vi "Unlock_project_folder.vi"() -> ()   [LabVIEW 2023]
uses:
  <vilib>/Utility/error.llb/Trim Whitespace One-Sided.vi
panel:
  out "status":string
  in  "stop":bool
  in  "File types":string="*.vi,*.vit,*.vim,*.ctl,*.ctt,*.lvlib,*.lvclass,*.xctl,*.xnode" caption="File types (comma separated)"
  out "File":path
  out "Slide":dbl(slide) scale=0.0..1.0
  out "Icon":picture
  in  "Output folder":path
  in  "Locked project folder":path
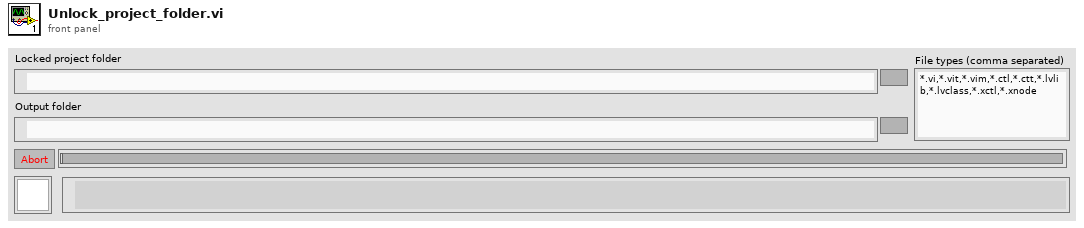
[diagram p1: front panel]
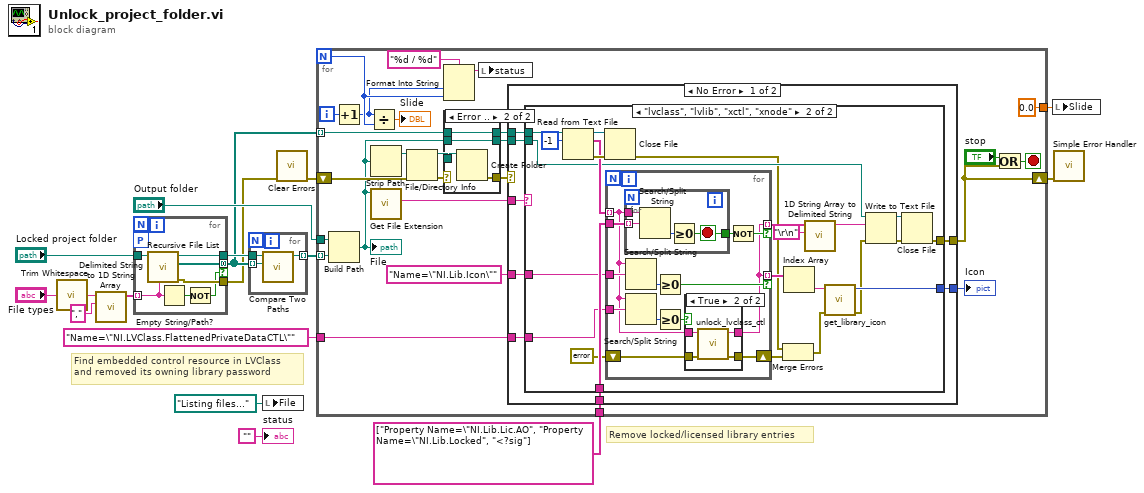
[diagram p0: block diagram]
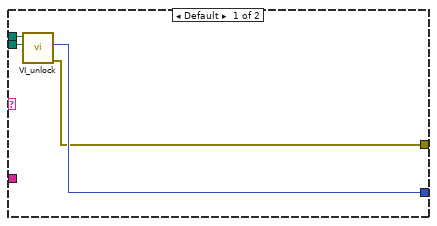
[diagram p3: hidden frame]
diagram:
  # "Remove locked/licensed library entries"
  # "Find embedded control resource in LVClass\nand removed its owning library password"
  n1 = call <vilib>:"Trim Whitespace.vi"("string"="File types") -> ("trimmed string"=w4:string)  [unwired: 1 in]
  n2 = call <vilib>:"Delimited String to 1D String Array.vi"("delimiter"="," ("delimiter (Tab)"), "delimited string"=w4) -> ("string array"=w3:string[])  [unwired: 9 in]
  n3 = for {
    tunnel: w3 -> [w20] mode=indexing
    workers-P: _ -> [_]
    tunnel: "Locked project folder" -> [w24]
    tunnel: [w23] -> w8 mode=concatenating if=w18
    tunnel: [w22] -> w7
    tunnel: [w21] -> w9
    n4 = call <vilib>:"Recursive File List.vi"("pattern"=w20, "Folder Path"=w24) -> ("error out"=w22:errorcluster, "All Files in Dir"=w23:path[], "dup Folder Path"=w21:path)  [unwired: 5 in, 2 out]
    n5 = Empty String/Path?(string/path=w20) -> (empty?=w19:bool)
    n6 = Not(x=w19) -> (.not. x?=w18:bool)
  }
  n7 = for {
    tunnel: w8 -> [w26] mode=indexing
    tunnel: w9 -> [w25]
    tunnel: [w27] -> w15 mode=indexing
    n8 = call <vilib>:"Compare Two Paths.vi"("Path 2"=w26, "Path 1"=w25) -> ("Relative Path from 1 to 2"=w27:path)  [unwired: 6 in, 3 out]
  }
  n9 = local write "File"(path "Listing files..." ("File")) -> ()
  n10 = call <vilib>:"Clear Errors.vi"("error in (no error)"=w7) -> ("error out"=w6:errorcluster)  [unwired: 5 in, 1 out]
  n11 = for {
    N -> [w31]
    tunnel: w8 -> [w39] mode=indexing
    tunnel: "Output folder" -> [w53]
    shift-right: [w34] -> w17
    shift-left: w6 -> [w48]
    tunnel: string[] ["Property Name=\"NI.Lib.Lic.AO", "Property Name=\"NI.Lib.Locked", "<?sig"] -> [w45]
    tunnel: w15 -> [w44] mode=indexing
    tunnel: "Name=\"NI.LVClass.FlattenedPrivateDataCTL\"" ("search string/char (-)") -> [w42]
    tunnel: [0.0] -> w12
    i -> [w50]
    stop <- w33 stop-if-true
    n12 = Build Path(base path=w53, name or relative path=w44) -> (appended path=w38:path)
    "File" <- w38
    n13 = Increment(x=w50) -> (x+1=w30:i32)
    n14 = Divide(x=w30, y=w31) -> (x/y=→"Slide":dbl)
    n15 = Strip Path(path=w38) -> (stripped path=w52:path)  [unwired: 1 out]
    n16 = call <vilib>:"Get File Extension.vi"("file"=w38) -> ("lowercase file extension"=w46:string)  [unwired: 6 in, 4 out]
    n17 = File/Directory Info(path=w52, error in=w48) -> (path out=w51:path, error out=w40:errorcluster)  [unwired: 5 out]
    n18 = Format Into String(format string="%d / %d", w30, w31) -> (resulting string=w28:string)  [unwired: 2 in, 1 out]
    n19 = case shown="Error .." w40 {
      selector: w40 -> [w56 _]
      tunnel: w51 -> [_ w60]
      tunnel: [w56 w59] -> w41
      tunnel: w39 -> [w54 w58]
      tunnel: w38 -> [w55 w57]
      tunnel: [w54 w58] -> w37
      tunnel: [w55 w57] -> w36
      frame No Error {
      }
      frame Error {
        n20 = Create Folder(path (use dialog)=w60) -> (error out=w59:errorcluster)  [unwired: 2 in, 2 out]
      }
    }
    n21 = local write "status"(w28) -> ()
    n22 = case shown="No Error" w41 {
      selector: w41 -> [_ w118]
      tunnel: w37 -> [w68 _]
      tunnel: w36 -> [w67 _]
      tunnel: [w66 _] -> w47
      tunnel: [w65 w118] -> w34
      tunnel: w46 -> [w64 _]
      tunnel: w45 -> [w63 _]
      tunnel: "Name=\"NI.Lib.Icon\"" ("search string/char (-)") -> [w62 _]
      tunnel: w42 -> [w61 _]
      frame No Error {
        n23 = case shown="\"lvclass\", \"lvlib\", \"xctl\", \"xnode\"" w64 {
          tunnel: w68 -> [w69 w87]
          tunnel: w67 -> [w72 w86]
          tunnel: [w71 w78] -> w66
          tunnel: [w70 w83] -> w65
          tunnel: w63 -> [_ w85]
          tunnel: w62 -> [_ w84]
          tunnel: w61 -> [_ w82]
          frame Default {
            n24 = call "VI_unlock.vi"("Output file"=w72, "Input file"=w69) -> ("error out"=w70:errorcluster, "Icon"=w71:picture)  [unwired: 5 in, 3 out]
          }
          frame "lvclass", "lvlib", "xctl", "xnode" {
            n25 = Read from Text File(file (use dialog)=w87, count=-1) -> (refnum out=w94:refnum<file>, text=w92:string[], error out=w95:errorcluster)  [unwired: 2 in, 1 out]
            n26 = Close File(refnum=w94, error in=w95) -> (error out=w79:errorcluster)  [unwired: 1 out]
            n27 = for {
              tunnel: w92 -> [w99] mode=indexing
              tunnel: w85 -> [w108]
              tunnel: [w98] -> w77 mode=indexing if=w106
              tunnel: w84 -> [w105]
              tunnel: [w98] -> w91 mode=indexing if=w103
              tunnel: w82 -> [w101]
              shift-right: [w97] -> w81
              shift-left: errorcluster {"status"=FALSE, "code"=0, "source"=""} ("error out") -> [w96]
              n28 = for {
                tunnel: w99 -> [w117]
                tunnel: w108 -> [w116] mode=indexing
                tunnel: [w114] -> w107
                stop <- w114 stop-if-true
                n29 = Search/Split String(string=w117, search string/char (-)=w116) -> (offset of match=w115:i32)  [unwired: 1 in, 2 out]
                n30 = Greater Or Equal To 0?(x=w115) -> (x >= 0?=w114:bool)
              }
              n31 = Search/Split String(string=w99, search string/char (-)=w105) -> (offset of match=w104:i32)  [unwired: 1 in, 2 out]
              n32 = Search/Split String(string=w99, search string/char (-)=w101) -> (offset of match=w102:i32)  [unwired: 1 in, 2 out]
              n33 = Greater Or Equal To 0?(x=w104) -> (x >= 0?=w103:bool)
              n34 = Greater Or Equal To 0?(x=w102) -> (x >= 0?=w100:bool)
              n35 = case shown="True" w100 {
                tunnel: w99 -> [w109 w113]
                tunnel: [w109 w112] -> w98
                tunnel: [_ w111] -> w97
                tunnel: w96 -> [_ w110]
                frame False {
                }
                frame True {
                  n36 = call "unlock_lvclass_ctl.vi"("error in (no error)"=w110, "Flattened\nPrivateDataCTL line"=w113) -> ("error out"=w111:errorcluster, "Unlocked Flattened CTL line"=w112:string)  [unwired: 8 in]
                }
              }
              n37 = Not(x=w107) -> (.not. x?=w106:bool)
            }
            n38 = Merge Errors(w79, w81) -> (w74:errorcluster)
            n39 = Index Array(array=w91) -> (element=w90:string)  [unwired: 1 in]
            n40 = call <vilib>:"1D String Array to Delimited String.vi"("delimiter"="\r\n", "string array"=w77) -> ("delimited string"=w75:string)  [unwired: 9 in]
            n41 = call "get_library_icon.vi"("error in (no error)"=w74, "Icon XML line"=w90) -> ("error out"=w73:errorcluster, "Icon"=w78:picture)  [unwired: 8 in]
            n42 = Write to Text File(file (use dialog)=w86, text=w75, error in=w73) -> (refnum out=w88:refnum<file>, error out=w89:errorcluster)  [unwired: 1 in, 1 out]
            n43 = Close File(refnum=w88, error in=w89) -> (error out=w83:errorcluster)  [unwired: 1 out]
          }
        }
      }
      frame Error {
      }
    }
    "Icon" <- w47
    n44 = Or(x="stop", y=w34) -> (x .or. y?=w33:bool)
  }
  n45 = local write "Slide"(w12) -> ()
  n46 = call <vilib>:"Simple Error Handler.vi"("error in (no error)"=w17) -> ()  [unwired: 4 in, 5 out]
  "status" <- ""
